vi "exchange rate_test.vi"() -> ()   [LabVIEW 2014]
uses:
  <vilib>/Utility/config.llb/Read Key (I32).vi
  <vilib>/Utility/config.llb/Read Key (String).vi
  <vilib>/Utility/config.llb/Write Key (String).vi
  <vilib>/Utility/config.llb/Write Key (I32).vi
  <vilib>/Utility/file.llb/Write To Spreadsheet File (string).vi
  <vilib>/regexp/Match Regular Expression.xnode
  <vilib>/httpClient/LabVIEWHTTPClient.lvlib
  <vilib>/Utility/config.llb/NI_LVConfig.lvlib
panel:
  out "부분이 삭제된 배열":string[](array[string])
  out "웨이브폼 그래프":i32[](graph)
  out "현재 환율 2":string
  in  "확인 버튼":bool
  in  "world":string(combo)="USD"
  in  "day":string(combo)="13"
  in  "month":string(combo)="08"
  in  "year":string(combo)="2018"
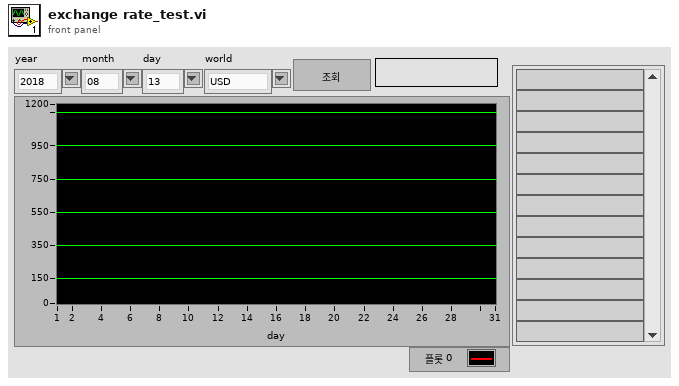
[diagram p1: front panel]
types:
  T1 = typedef "NI_LVConfig.lvlib/Config Data RefNum.ctl" = refnum<k1>
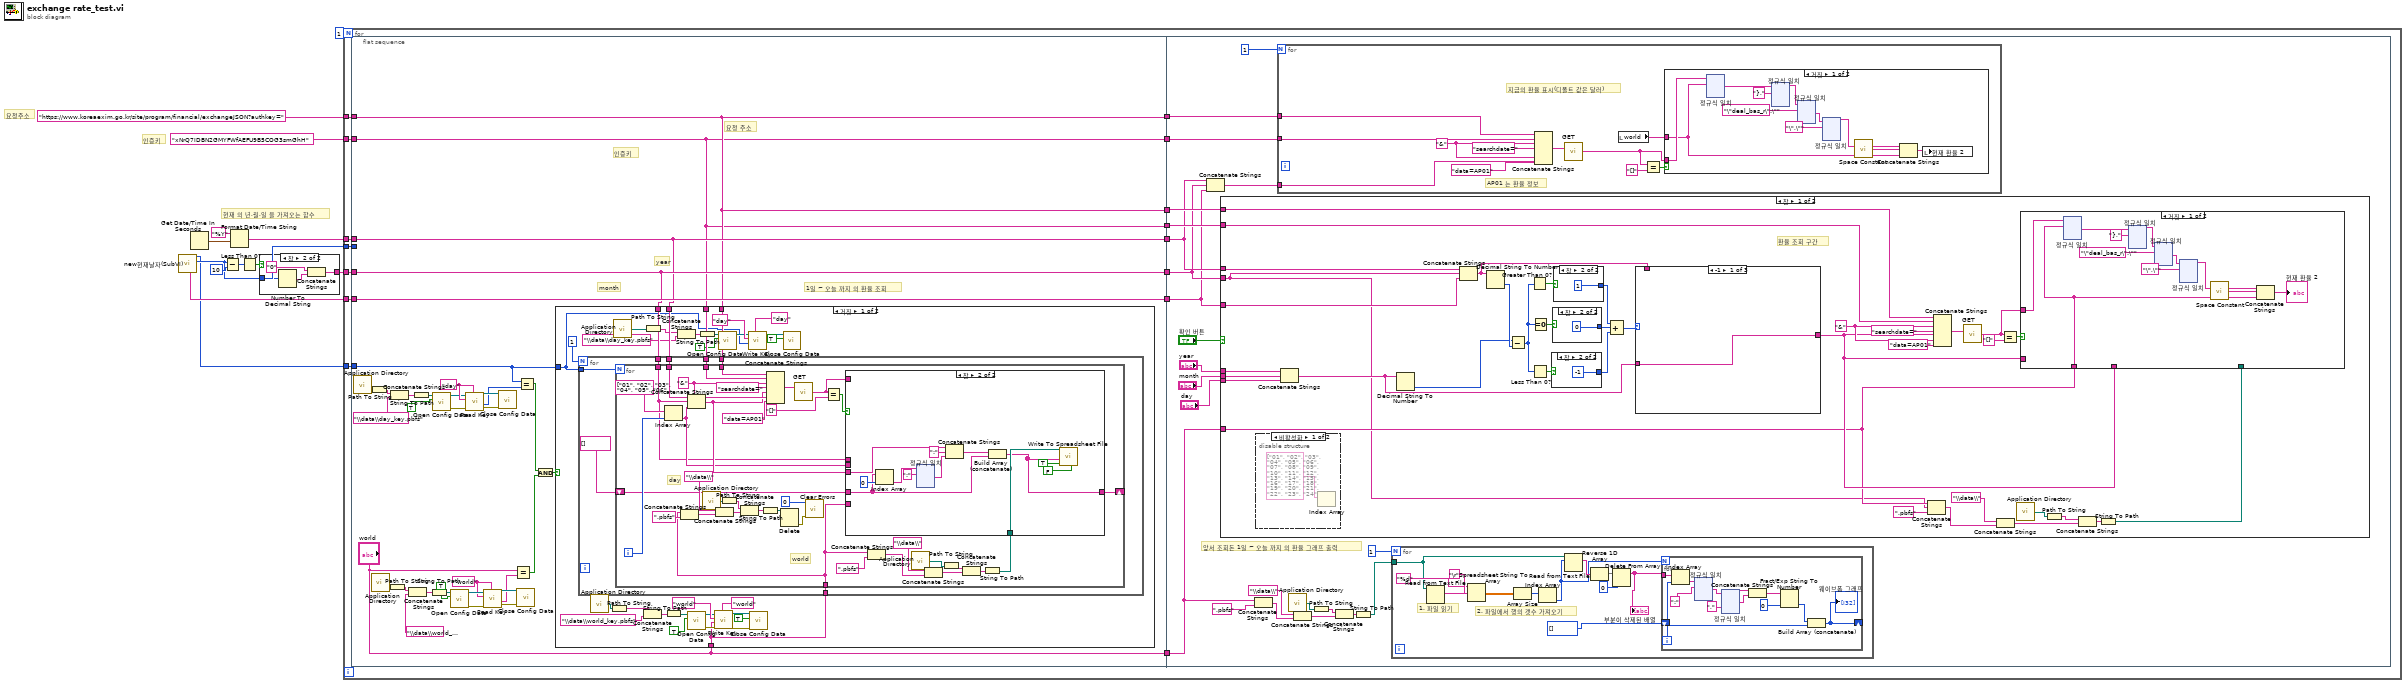
[diagram p0: block diagram]
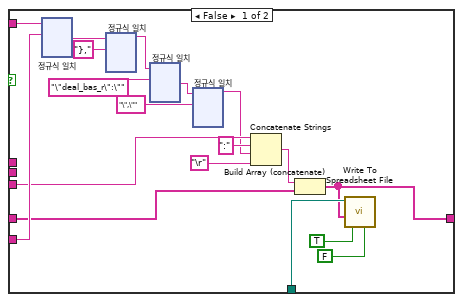
[diagram p2: hidden frame]
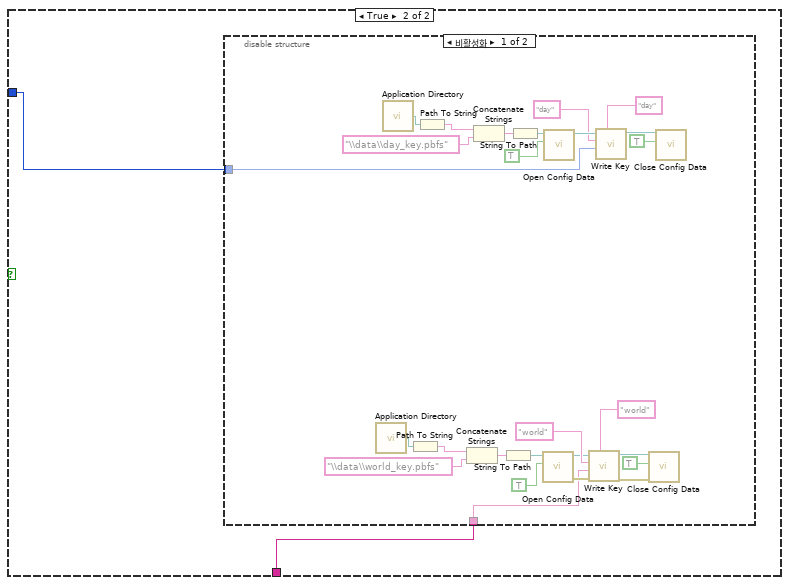
[diagram p3: hidden frame]
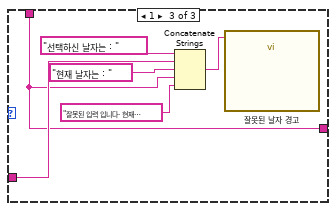
[diagram p8: hidden frame]
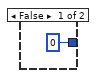
[diagram p9: hidden frame]
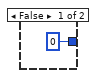
[diagram p10: hidden frame]
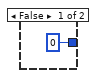
[diagram p11: hidden frame]
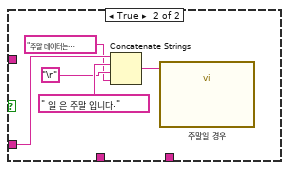
[diagram p12: hidden frame]
diagram:
  # "인증키"
  # "요청주소"
  # "현재 의 년,월,일 을 가져오는 함수"
  n1 = call "new현재날자(SubVI).vi"() -> ("월"=w7:i32, "일"=w3:i32, "일 문자열"=w6:string)  [unwired: 5 in, 4 out]
  n2 = Get Date/Time In Seconds() -> (seconds since 1Jan1904=w10:timestamp)
  n3 = Subtract(x=w7, y=10) -> (x-y=w12:i32)
  n4 = Format Date/Time String(time format string (%c)="%Y" ("시간 포맷 문자열 (%c)"), seconds (now)=w10) -> (date/time string=w8:string)  [unwired: 1 in]
  n5 = Less Than 0?(x=w12) -> (x < 0?=w11:bool)
  n6 = case shown="참" w11 {
    tunnel: w7 -> [_ w17]
    tunnel: [_ w14] -> w1
    frame False {
    }
    frame True {
      n7 = Number To Decimal String(number=w17) -> (decimal integer string=w16:string)  [unwired: 1 in]
      n8 = Concatenate Strings("0", w16) -> (w14:string)
    }
  }
  n9 = for {
    N: 1 -> [_]
    tunnel: w8 -> [w29]
    tunnel: w7 -> [w28]
    tunnel: w6 -> [w26]
    tunnel: w1 -> [w27]
    tunnel: "https://www.koreaexim.go.kr/site/program/financial/exchangeJSON?authkey=" -> [w31]
    tunnel: "xNrQ7IDBN2GMYFWfAEFU9B5COG3smGhH" -> [w30]
    tunnel: w3 -> [w32]
    n10 = flat-sequence {
      tunnel: w32 -> [w39]
      tunnel: w31 -> [w35]
      tunnel: w30 -> [w34]
      tunnel: w29 -> [w36]
      tunnel: w28 -> [_]
      tunnel: w27 -> [w37]
      tunnel: w26 -> [w38]
      tunnel: ["world"] -> w25
      tunnel: [w35] -> w24
      tunnel: [w34] -> w23
      tunnel: [w36] -> w22
      tunnel: [w37] -> w21
      tunnel: [w38] -> w20
      tunnel: [w35] -> w19
      tunnel: [w34] -> w18
      tunnel: w25 -> [w776]
      tunnel: w24 -> [w775]
      tunnel: w23 -> [w774]
      tunnel: w22 -> [w771]
      tunnel: w21 -> [w770]
      tunnel: w20 -> [w769]
      tunnel: w19 -> [w773]
      tunnel: w18 -> [w772]
      frame #0 {
        w46 = "world" ("key")
        w66 = "day" ("key")
        # "1일 ~ 오늘 까지 의 환율 조회"
        # "year"
        # "month"
        # "요청 주소"
        # "인증키"
        n11 = call <vilib>:"Application Directory.vi"() -> ("Application Directory"=w62:path)
        n12 = Path To String(path=w62) -> (string=w64:string)
        n13 = call <vilib>:"Application Directory.vi"() -> ("Application Directory"=w50:path)
        n14 = Path To String(path=w50) -> (string=w48:string)
        n15 = Concatenate Strings(w64, "\\data\\day_key.pbfs" ("문자열")) -> (w63:string)
        n16 = Concatenate Strings(w48, "\\data\\world_key.pbfs" ("문자열")) -> (w49:string)
        n17 = String To Path(string=w63) -> (path=w65:path)
        n18 = String To Path(string=w49) -> (path=w47:path)
        n19 = call <vilib>:"Open Config Data.vi"("create file if necessary (T)"=TRUE, "configuration file path"=w65) -> ("error out"=w58:errorcluster, "refnum"=w57:T1)  [unwired: 7 in, 1 out]
        n20 = call <vilib>:"Open Config Data.vi"("create file if necessary (T)"=TRUE, "configuration file path"=w47) -> ("error out"=w54:errorcluster, "refnum"=w55:T1)  [unwired: 7 in, 1 out]
        n21 = call-poly <vilib>:"Read Key.vi"("section"=w66, "error in (no error)"=w58, "key"=w66, "refnum"=w57) -> ("error out"=w59:errorcluster, "value"=w56:i32, "refnum out"=w60:T1)  [unwired: 4 in, 1 out]
        n22 = call-poly <vilib>:"Read Key.vi"("section"=w46, "error in (no error)"=w54, "key"=w46, "refnum"=w55) -> ("error out"=w53:errorcluster, "value"=w45:string, "refnum out"=w52:T1)  [unwired: 4 in, 1 out]
        n23 = call <vilib>:"Close Config Data.vi"("error in (no error)"=w59, "refnum"=w60) -> ()  [unwired: 8 in, 2 out]
        n24 = Equal?(x="world", y=w45) -> (x = y?=w43:bool)
        n25 = call <vilib>:"Close Config Data.vi"("error in (no error)"=w53, "refnum"=w52) -> ()  [unwired: 8 in, 2 out]
        n26 = Equal?(x=w39, y=w56) -> (x = y?=w44:bool)
        n27 = And(x=w44, y=w43) -> (x .and. y?=w42:bool)
        n28 = case shown="거짓" w42 {
          tunnel: w39 -> [w81 w741]
          tunnel: w36 -> [w97 _]
          tunnel: w35 -> [w96 _]
          tunnel: w34 -> [w95 _]
          tunnel: w37 -> [w94 _]
          tunnel: "world" -> [w67 w742]
          frame False {
            n29 = for {
              N: 1 -> [_]
              tunnel: w81 -> [w104]
              tunnel: w97 -> [w103]
              tunnel: w96 -> [w102]
              tunnel: w95 -> [w101]
              tunnel: w94 -> [w100]
              tunnel: w67 -> [w99]
              n30 = for {
                N: w104 -> [_]
                tunnel: w103 -> [w135]
                tunnel: w102 -> [w137]
                tunnel: w101 -> [w136]
                tunnel: w100 -> [w120]
                tunnel: w99 -> [w107]
                shift-right: [w105] -> _
                shift-left: string[] [] -> [w106]
                i -> [w134]
                w139 = "&" ("문자열")
                # "day"
                # "world"
                n31 = Index Array(array=string[] ["01", "02", "03", "04", "05", "06", "07", "08", "09", "10", "11", "12", "13", "14", "15", "16", "17", "18", "19", "20", "21", "22", "23", "24", "25", "26", "27", "28", "29", "30", "31"], index=w134) -> (element=w127:string)
                n32 = Concatenate Strings(w107, ".pbfs" ("문자열")) -> (w110:string)
                n33 = Concatenate Strings(w135, w120, w127) -> (w129:string)
                n34 = call <vilib>:"Application Directory.vi"() -> ("Application Directory"=w112:path)
                n35 = Concatenate Strings("\\data\\" ("문자열"), w110) -> (w109:string)
                n36 = Path To String(path=w112) -> (string=w114:string)
                n37 = Concatenate Strings(w114, w109) -> (w113:string)
                n38 = String To Path(string=w113) -> (path=w115:path)
                n39 = Concatenate Strings(w137, w136, w139, "searchdate=" ("문자열"), w129, w139, "data=AP01" ("문자열")) -> (w132:string)
                n40 = Delete(path (use dialog)=w115) -> (error out=w117:errorcluster)  [unwired: 4 in, 2 out]
                n41 = call <vilib>:"GET.vi"("url"=w132) -> ("body"=w130:string)  [unwired: 11 in, 3 out]
                n42 = call <vilib>:"Clear Errors.vi"("error in (no error)"=w117, "specific error code to clear (0: all)"=0) -> ()  [unwired: 4 in, 2 out]
                n43 = Equal?(x=w130, y="[]") -> (x = y?=w131:bool)
                n44 = Concatenate Strings(w107, ".pbfs" ("문자열")) -> (w122:string)
                n45 = call <vilib>:"Application Directory.vi"() -> ("Application Directory"=w124:path)
                n46 = Concatenate Strings("\\data\\" ("문자열"), w122) -> (w121:string)
                n47 = Path To String(path=w124) -> (string=w126:string)
                n48 = Concatenate Strings(w126, w121) -> (w125:string)
                n49 = String To Path(string=w125) -> (path=w119:path)
                n50 = case shown="참" w131 {
                  tunnel: w129 -> [w150 w626]
                  tunnel: w130 -> [w152 _]
                  tunnel: w107 -> [w151 _]
                  tunnel: w120 -> [_ _]
                  tunnel: w127 -> [_ _]
                  tunnel: w119 -> [w147 w625]
                  tunnel: w106 -> [w144 w618]
                  tunnel: [w142 w619] -> w105
                  frame False {
                    n51 = xnode ("정규식 일치")("입력 문자열"=w152, "정규식"=w151) -> ("일치 구문 뒤"=w153:string)  [unwired: 4 in, 4 out]
                    n52 = xnode ("정규식 일치")("입력 문자열"=w153, "정규식"="},") -> ("일치 구문 앞"=w155:string)  [unwired: 4 in, 4 out]
                    n53 = xnode ("정규식 일치")("입력 문자열"=w155, "정규식"="\"deal_bas_r\":\"") -> ("일치 구문 뒤"=w157:string)  [unwired: 4 in, 4 out]
                    n54 = xnode ("정규식 일치")("입력 문자열"=w157, "정규식"="\",\"") -> ("일치 구문 앞"=w148:string)  [unwired: 4 in, 4 out]
                    n55 = Concatenate Strings(w150, ":" ("문자열"), w148, "\r") -> (w143:string)
                    n56 = Build Array (concatenate)(w143, w144) -> (w142:string[])
                    n57 = call-poly <vilib>:"Write To Spreadsheet File.vi"("transpose? (no:F)"=FALSE, "append to file? (new file:F)"=TRUE, "1D data"=w142, "file path (dialog if empty)"=w147) -> ()  [unwired: 4 in, 1 out]
                  }
                  frame True {
                    n58 = Index Array(array=w618, index=0 ("인덱스")) -> (element=w617:string)
                    n59 = xnode "정규식 일치"("입력 문자열"=w617, "정규식"=":") -> ("일치 구문 뒤"=w615:string)  [unwired: 4 in, 4 out]
                    n60 = Concatenate Strings(w626, ":", w615) -> (w621:string)
                    n61 = Build Array (concatenate)(w621, w618) -> (w619:string[])
                    n62 = call-poly <vilib>:"Write To Spreadsheet File.vi"("transpose? (no:F)"=FALSE, "append to file? (new file:F)"=TRUE, "1D data"=w619, "file path (dialog if empty)"=w625) -> ()  [unwired: 4 in, 1 out]
                  }
                }
              }
            }
            n63 = call <vilib>:"Application Directory.vi"() -> ("Application Directory"=w77:path)
            n64 = Path To String(path=w77) -> (string=w79:string)
            n65 = call <vilib>:"Application Directory.vi"() -> ("Application Directory"=w88:path)
            n66 = Concatenate Strings(w79, "\\data\\world_key.pbfs" ("문자열")) -> (w78:string)
            n67 = Path To String(path=w88) -> (string=w90:string)
            n68 = String To Path(string=w78) -> (path=w80:path)
            n69 = Concatenate Strings(w90, "\\data\\day_key.pbfs" ("문자열")) -> (w89:string)
            n70 = call <vilib>:"Open Config Data.vi"("create file if necessary (T)"=TRUE, "configuration file path"=w80) -> ("error out"=w69:errorcluster, "refnum"=w70:T1)  [unwired: 7 in, 1 out]
            n71 = String To Path(string=w89) -> (path=w91:path)
            n72 = call-poly <vilib>:"Write Key.vi"("section"="world", "error in (no error)"=w69, "value"=w67, "key"="world", "refnum"=w70) -> ("error out"=w72:errorcluster, "refnum out"=w71:T1)  [unwired: 4 in, 1 out]
            n73 = call <vilib>:"Open Config Data.vi"("create file if necessary (T)"=TRUE, "configuration file path"=w91) -> ("refnum"=w82:T1)  [unwired: 7 in, 2 out]
            n74 = call-poly <vilib>:"Write Key.vi"("section"="day", "value"=w81, "key"="day", "refnum"=w82) -> ("refnum out"=w83:T1)  [unwired: 5 in, 2 out]
            n75 = call <vilib>:"Close Config Data.vi"("error in (no error)"=w72, "write file if changed (T)"=TRUE, "refnum"=w71) -> ()  [unwired: 7 in, 2 out]
            n76 = call <vilib>:"Close Config Data.vi"("write file if changed (T)"=TRUE, "refnum"=w83) -> ()  [unwired: 8 in, 2 out]
          }
          frame True {
            n77 = disable-structure shown="비활성화" {
              disable-tunnel: w742 -> [w744 _]
              disable-tunnel: w741 -> [w743 _]
              frame Disabled {
                n78 = call <vilib>:"Application Directory.vi"() -> ("Application Directory"=w765:path)
                n79 = call <vilib>:"Application Directory.vi"() -> ("Application Directory"=w750:path)
                n80 = Path To String(path=w765) -> (string=w767:string)
                n81 = Path To String(path=w750) -> (string=w748:string)
                n82 = Concatenate Strings(w767, "\\data\\world_key.pbfs" ("문자열")) -> (w766:string)
                n83 = Concatenate Strings(w748, "\\data\\day_key.pbfs" ("문자열")) -> (w749:string)
                n84 = String To Path(string=w766) -> (path=w768:path)
                n85 = String To Path(string=w749) -> (path=w747:path)
                n86 = call <vilib>:"Open Config Data.vi"("create file if necessary (T)"=TRUE, "configuration file path"=w768) -> ("error out"=w757:errorcluster, "refnum"=w758:T1)  [unwired: 7 in, 1 out]
                n87 = call <vilib>:"Open Config Data.vi"("create file if necessary (T)"=TRUE, "configuration file path"=w747) -> ("refnum"=w756:T1)  [unwired: 7 in, 2 out]
                n88 = call-poly <vilib>:"Write Key.vi"("section"="world", "error in (no error)"=w757, "value"=w744, "key"="world", "refnum"=w758) -> ("error out"=w760:errorcluster, "refnum out"=w759:T1)  [unwired: 4 in, 1 out]
                n89 = call-poly <vilib>:"Write Key.vi"("section"="day", "value"=w743, "key"="day", "refnum"=w756) -> ("refnum out"=w755:T1)  [unwired: 5 in, 2 out]
                n90 = call <vilib>:"Close Config Data.vi"("error in (no error)"=w760, "write file if changed (T)"=TRUE, "refnum"=w759) -> ()  [unwired: 7 in, 2 out]
                n91 = call <vilib>:"Close Config Data.vi"("write file if changed (T)"=TRUE, "refnum"=w755) -> ()  [unwired: 8 in, 2 out]
              }
              frame Enabled {
              }
            }
          }
        }
      }
      frame #1 {
        # "앞서 조회돈 1일 ~ 오늘 까지 의 환율 그래프 출력"
        n92 = Concatenate Strings(w771, w770, w769) -> (w778:string)
        n93 = case shown="참" "확인 버튼" {
          tunnel: w776 -> [w1532 _]
          tunnel: w769 -> [w1531 _]
          tunnel: w771 -> [w1530 _]
          tunnel: w770 -> [w1523 _]
          tunnel: "month" -> [w1527 _]
          tunnel: "day" -> [w1528 _]
          tunnel: "year" -> [w1526 _]
          tunnel: w773 -> [w1525 _]
          tunnel: w772 -> [w1524 _]
          frame True {
            w1558 = "&" ("문자열")
            # "환율 조회 구간"
            n94 = disable-structure shown="비활성화" {
              frame Disabled {
                n95 = Index Array(array=string[] ["01", "02", "03", "04", "05", "06", "07", "08", "09", "10", "11", "12", "13", "14", "15", "16", "17", "18", "19", "20", "21", "22", "23", "24", "25", "26", "27", "28", "29", "30", "31"]) -> ()  [unwired: 1 in, 1 out]
              }
              frame Enabled {
              }
            }
            n96 = Concatenate Strings(w1526, w1527, w1528) -> (w1529:string)
            n97 = Decimal String To Number(string=w1529) -> (number=w1551:i32)  [unwired: 2 in, 1 out]
            n98 = Concatenate Strings(w1530, w1523, w1531) -> (w1542:string)
            n99 = Decimal String To Number(string=w1542) -> (number=w1552:i32)  [unwired: 2 in, 1 out]
            n100 = Subtract(x=w1551, y=w1552) -> (x-y=w1547:i32)
            n101 = Greater Than 0?(x=w1547) -> (x > 0?=w1548:bool)
            n102 = Less Than 0?(x=w1547) -> (x < 0?=w1550:bool)
            n103 = Equal To 0?(x=w1547) -> (x = 0?=w1549:bool)
            n104 = case shown="참" w1550 {
              tunnel: [0 -1] -> w1544
              frame False {
              }
              frame True {
              }
            }
            n105 = case shown="참" w1549 {
              tunnel: [0 0] -> w1545
              frame False {
              }
              frame True {
              }
            }
            n106 = case shown="참" w1548 {
              tunnel: [0 1] -> w1546
              frame False {
              }
              frame True {
              }
            }
            n107 = Compound Arithmetic op=ADD(w1546, w1545, w1544) -> (w1543:i32)
            n108 = case shown="-1" w1543 {
              tunnel: w1529 -> [w1561 _ w1567]
              tunnel: w1542 -> [_ w1562 w1565]
              tunnel: [w1561 w1562 w1565] -> w1534
              frame -1 {
              }
              frame 0, Default {
              }
              frame 1 {
                n109 = Concatenate Strings("선택하신 날자는 : " ("문자열"), w1567, "현재 날자는 : ", w1565, "잘못된 입력 입니다. 현재 날자로 검색을 진행 합니다." ("문자열")) -> (w1563:string)
                n110 = call "잘못된 날자 경고"("Message"=w1563) -> ()  [unwired: 9 in, 2 out]
              }
            }
            n111 = Concatenate Strings(w1532, w1523, ".pbfs" ("문자열")) -> (w1536:string)
            n112 = Concatenate Strings(w1525, w1524, w1558, "searchdate=" ("문자열"), w1534, w1558, "data=AP01" ("문자열")) -> (w1556:string)
            n113 = call <vilib>:"GET.vi"("url"=w1556) -> ("body"=w1553:string)  [unwired: 11 in, 3 out]
            n114 = Concatenate Strings("\\data\\" ("문자열"), w1536) -> (w1535:string)
            n115 = Equal?(x=w1553, y="[]") -> (x = y?=w1554:bool)
            n116 = call <vilib>:"Application Directory.vi"() -> ("Application Directory"=w1539:path)
            n117 = Path To String(path=w1539) -> (string=w1541:string)
            n118 = Concatenate Strings(w1541, w1535) -> (w1540:string)
            n119 = String To Path(string=w1540) -> (path=w1533:path)
            n120 = case shown="거짓" w1554 {
              tunnel: w1534 -> [_ w2046]
              tunnel: w1553 -> [w1577 _]
              tunnel: w1532 -> [w1576 _]
              tunnel: w1534 -> [_ _]
              tunnel: w1533 -> [_ _]
              frame False {
                n121 = xnode ("정규식 일치")("입력 문자열"=w1577, "정규식"=w1576) -> ("일치 구문 뒤"=w1578:string)  [unwired: 4 in, 4 out]
                n122 = xnode ("정규식 일치")("입력 문자열"=w1578, "정규식"="},") -> ("일치 구문 앞"=w1580:string)  [unwired: 4 in, 4 out]
                n123 = xnode ("정규식 일치")("입력 문자열"=w1580, "정규식"="\"deal_bas_r\":\"") -> ("일치 구문 뒤"=w1582:string)  [unwired: 4 in, 4 out]
                n124 = xnode ("정규식 일치")("입력 문자열"=w1582, "정규식"="\",\"") -> ("일치 구문 앞"=w1575:string)  [unwired: 4 in, 4 out]
                n125 = call <vilib>:"Space Constant.vi"() -> ("String"=w1584:string)
                n126 = Concatenate Strings(w1575, w1584, w1576) -> (→"현재 환율 2":string)
              }
              frame True {
                n127 = Concatenate Strings(w2046, " 일 은 주말 입니다.", "\r", "주말 데이터는 제공되지 않습니다.") -> (w2042:string)
                n128 = call "주말일 경우"("Message"=w2042) -> ()  [unwired: 9 in, 2 out]
              }
            }
          }
          frame False {
          }
        }
        n129 = Concatenate Strings(w776, ".pbfs" ("문자열")) -> (w785:string)
        n130 = for {
          N: 1 -> [_]
          tunnel: w778 -> [w1051]
          tunnel: w775 -> [w1046]
          tunnel: w774 -> [w1045]
          w1053 = "&" ("문자열")
          # "지금의 환율 표시(디폴트 값은 달러)"
          # "AP01 는 환율 정보"
          n131 = Concatenate Strings(w1046, w1045, w1053, "searchdate=" ("문자열"), w1051, w1053, "data=AP01" ("문자열")) -> (w1055:string)
          n132 = call <vilib>:"GET.vi"("url"=w1055) -> ("body"=w1047:string)  [unwired: 11 in, 3 out]
          n133 = local read "world"() -> (w1050:string)
          n134 = Equal?(x=w1047, y="[]") -> (x = y?=w1048:bool)
          n135 = case shown="거짓" w1048 {
            tunnel: w1047 -> [w1059 _]
            tunnel: w1050 -> [w1057 _]
            frame False {
              n136 = xnode ("정규식 일치")("입력 문자열"=w1059, "정규식"=w1057) -> ("일치 구문 뒤"=w1060:string)  [unwired: 4 in, 4 out]
              n137 = xnode ("정규식 일치")("입력 문자열"=w1060, "정규식"="},") -> ("일치 구문 앞"=w1062:string)  [unwired: 4 in, 4 out]
              n138 = xnode ("정규식 일치")("입력 문자열"=w1062, "정규식"="\"deal_bas_r\":\"") -> ("일치 구문 뒤"=w1064:string)  [unwired: 4 in, 4 out]
              n139 = xnode ("정규식 일치")("입력 문자열"=w1064, "정규식"="\",\"") -> ("일치 구문 앞"=w1058:string)  [unwired: 4 in, 4 out]
              n140 = call <vilib>:"Space Constant.vi"() -> ("String"=w1066:string)
              n141 = Concatenate Strings(w1058, w1066, w1057) -> (w1056:string)
              n142 = local write "현재 환율 2"(w1056) -> ()
            }
            frame True {
            }
          }
        }
        n143 = call <vilib>:"Application Directory.vi"() -> ("Application Directory"=w788:path)
        n144 = Concatenate Strings("\\data\\" ("문자열"), w785) -> (w784:string)
        n145 = Path To String(path=w788) -> (string=w790:string)
        n146 = Concatenate Strings(w790, w784) -> (w789:string)
        n147 = String To Path(string=w789) -> (path=w791:path)
        n148 = for {
          N: 1 -> [_]
          tunnel: w791 -> [w798]
          # "2. 파일에서 행의 갯수 가져오기"
          # "1. 파일 읽기"
          n149 = Read from Text File(file (use dialog)=w798) -> (text=w803:string)  [unwired: 1 in, 5 out]
          n150 = Spreadsheet String To Array(delimiter (Tab)="\r", format string="%d", spreadsheet string=w803) -> (array=w801:dbl[][])  [unwired: 1 out]
          n151 = Array Size(array=w801) -> (size(s)=w802:i32[])
          n152 = Index Array(array=w802) -> (element=w795:i32)  [unwired: 1 in]
          n153 = Read from Text File(file (use dialog)=w798, count=w795) -> (text=w796:string[])  [unwired: 1 in, 4 out]
          n154 = Reverse 1D Array(array=w796) -> (reversed array=w794:string[])
          n155 = Delete From Array(array=w794, index=0 ("인덱스")) -> (array with subset deleted=w793:string[])  [unwired: 1 in, 1 out]
          "부분이 삭제된 배열" <- w793
          n156 = for {
            N: w795 -> [_]
            tunnel: w793 -> [w810]
            shift-right: [w808] -> _
            shift-left: i32[] [] -> [w809]
            i -> [w811]
            n157 = Index Array(array=w810, index=w811) -> (element=w816:string)
            n158 = xnode "정규식 일치"("입력 문자열"=w816, "정규식"=":") -> ("일치 구문 뒤"=w807:string)  [unwired: 4 in, 4 out]
            n159 = xnode "정규식 일치"("입력 문자열"=w807, "정규식"=",") -> ("일치 구문 앞"=w813:string, "일치 구문 뒤"=w812:string)  [unwired: 4 in, 3 out]
            n160 = Concatenate Strings(w813, w812) -> (w806:string)
            n161 = Fract/Exp String To Number(string=w806, default (0 dbl)=0) -> (number=w805:i32)  [unwired: 2 in, 1 out]
            n162 = Build Array (concatenate)(w805, w809) -> (w808:i32[])
            "웨이브폼 그래프" <- w808
          }
        }
      }
    }
  }
